vi "get desired keys.vi"(8 "error in":errorcluster, 11 "fixed channel configuration in":refnum<class "control module configuration.lvclass">) -> (0 "error out":errorcluster, 2 "desired keys":string[](array[string]), 3 "fixed channel configuration out":refnum<class "control module configuration.lvclass">)   [LabVIEW 2013, in "control module configuration.lvclass"]
uses:
  control module configuration.lvclass
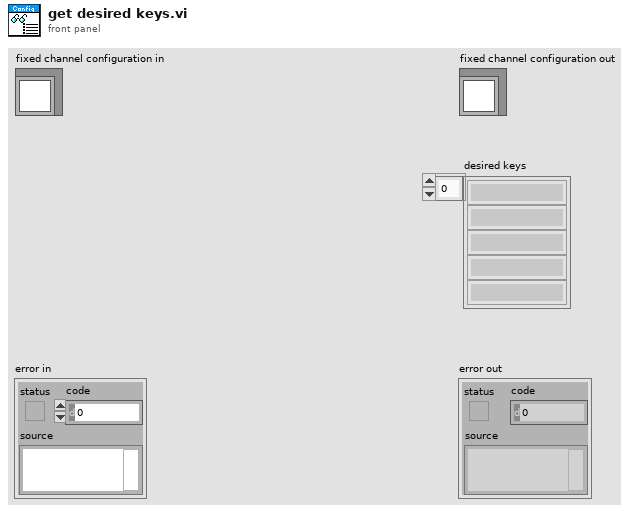
[diagram p1: front panel]
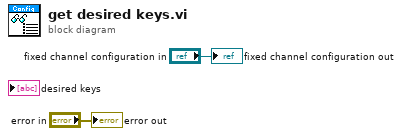
[diagram p0: block diagram]
diagram:
  "error out" <- "error in"
  "fixed channel configuration out" <- "fixed channel configuration in"
